vi "读取自定义数据.vi"() -> ()   [LabVIEW 2018]
uses:
  <vilib>/vision/Image Controls.llb/Vision Info Type2.ctl
  <vilib>/vision/Image Controls.llb/IMAQ Image.ctl
  <vilib>/vision/NI_Vision_Development_Module.lvlib
panel:
  out "error out":errorcluster
  out "Keys":string[](array[string])
  out "Custom Data Out":string
  out "Present?":bool=TRUE
  in  "error in (no error)":errorcluster
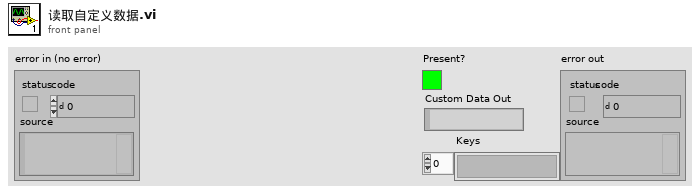
[diagram p1: front panel]
types:
  T1 = typedef "IMAQ Image.ctl" = refnum<image>
  T2 = typedef "Vision Info Type2.ctl" = u32
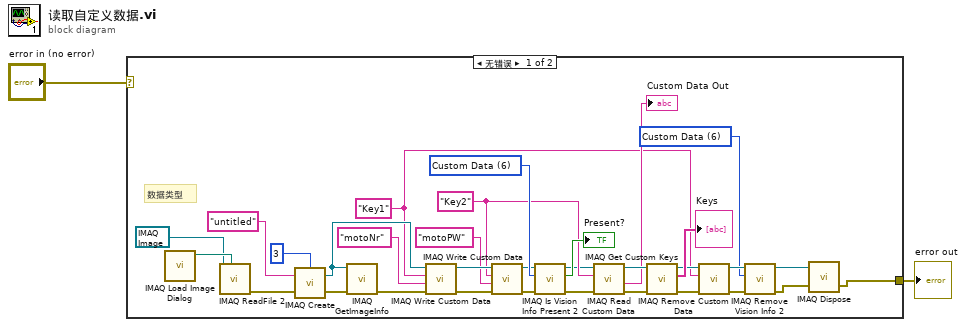
[diagram p0: block diagram]
diagram:
  n1 = case shown="无错误" "error in (no error)" {
    selector: "error in (no error)" -> [_ w35]
    tunnel: [w4 w35] -> w1
    frame No Error {
      w7 = T2 6 items=["Any", "Calibration", "Overlay", "Grayscale Template", "Color Template", "Geometric Template", "Custom Data", "Golden Template", "Geometric Template 2", "Contour Data", "Camera Model", "Pyramid Grayvalue Template", "Pyramid Gradient Template"] ("Vision Info")
      w23 = T2 6 items=["Any", "Calibration", "Overlay", "Grayscale Template", "Color Template", "Geometric Template", "Custom Data", "Golden Template", "Geometric Template 2", "Contour Data", "Camera Model", "Pyramid Grayvalue Template", "Pyramid Gradient Template"] ("Vision Info")
      w18 = "Key2" ("Key")
      w10 = "Key1" ("Key")
      # "数据类型"
      n2 = call "IMAQ Load Image Dialog"() -> ("Path"=w33:path)  [unwired: 9 in, 2 out]
      n3 = call "IMAQ ReadFile 2"("File Path"=w33, "Image"=T1 refnum) -> ("error out"=w34:errorcluster)  [unwired: 5 in, 4 out]
      n4 = call "IMAQ Create"("Border Size"=3, "Image Name"="untitled", "error in (no error)"=w34) -> ("New Image"=w29:T1, "error out"=w30:errorcluster)  [unwired: 2 in]
      n5 = call "IMAQ GetImageInfo"("error in (no error)"=w30, "Image"=w29) -> ("error out"=w28:errorcluster)  [unwired: 2 in, 7 out]
      n6 = call "IMAQ Write Custom Data"("error in (no error)"=w28, "Custom Data In"="motoNr", "Key"=w10, "Image"=w29) -> ("error out"=w25:errorcluster, "Image Out"=w26:T1)  [unwired: 6 in]
      n7 = call "IMAQ Write Custom Data"("error in (no error)"=w25, "Custom Data In"="motoPW", "Key"=w18, "Image"=w26) -> ("error out"=w22:errorcluster, "Image Out"=w21:T1)  [unwired: 6 in]
      n8 = call "IMAQ Is Vision Info Present 2"("error in (no error)"=w22, "Vision Info"=w23, "Image"=w21) -> ("error out"=w19:errorcluster, "Present?"=→"Present?":bool, "Image (duplicate)"=w17:T1)  [unwired: 6 in]
      n9 = call "IMAQ Read Custom Data"("error in (no error)"=w19, "Key"=w18, "Image"=w17) -> ("error out"=w15:errorcluster, "Custom Data Out"=→"Custom Data Out":string, "Image (duplicate)"=w16:T1)  [unwired: 6 in]
      n10 = call "IMAQ Get Custom Keys"("error in (no error)"=w15, "Image"=w16) -> ("error out"=w11:errorcluster, "Keys"=→"Keys":string[], "Image (duplicate)"=w12:T1)  [unwired: 6 in, 1 out]
      n11 = call "IMAQ Remove Custom Data"("error in (no error)"=w11, "Key"=w10, "Image"=w12) -> ("error out"=w8:errorcluster, "Image Out"=w9:T1)  [unwired: 6 in, 1 out]
      n12 = call "IMAQ Remove Vision Info 2"("error in (no error)"=w8, "Vision Info"=w7, "Image"=w9) -> ("error out"=w5:errorcluster, "Image Out"=w6:T1)  [unwired: 7 in]
      n13 = call "IMAQ Dispose"("Image"=w6, "error in (no error)"=w5) -> ("error out"=w4:errorcluster)  [unwired: 4 in]
    }
    frame Error {
    }
  }
  "error out" <- w1
